vi "Load Sound Player.vi"(10 "Select sound player:":T1=1 items=["Sound Card", "Sound Visualizer"]) -> (0 "error out":errorcluster, 3 "Sound Player out":refnum<class "Sound Player.lvclass">)   [LabVIEW 2010, in "Sound Demo.lvclass"]
doc: "Dynamically load either Sound Visualizer or Sound Card.lvclass based on user input.\n\nBuild the path to the class using the string values of the Select sound player: ring control."
uses:
  Sound Demo.lvclass
  Select Sound Player.ctl
  Sound Player/Sound Player.lvclass
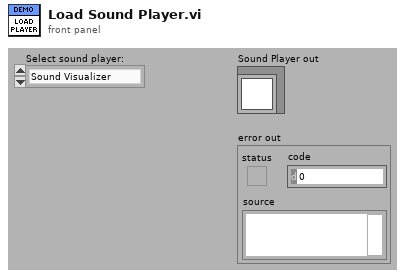
[diagram p1: front panel]
types:
  T1 = typedef "Sound Demo.lvclass/Select Sound Player.ctl" = u16
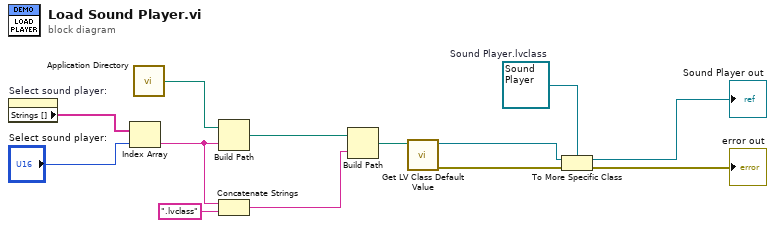
[diagram p0: block diagram]
diagram:
  w10 = refnum<class "Sound Player.lvclass"> refnum  # Sound Player.lvclass
  n1 = property on="Select sound player:" class="Ring (strict)"() -> ("Strings []"=w7:string[])  [unwired: 2 in, 2 out]
  n2 = Index Array "Index Array"(array=w7, index="Select sound player:") -> (element=w1:string)
  n3 = call <vilib>:"Application Directory.vi"() -> ("Application Directory"=w4:path)
  n4 = Build Path(base path=w4, name or relative path=w1) -> (appended path=w2:path)
  n5 = Concatenate Strings "Concatenate Strings"(w1, ".lvclass" ("string")) -> (w3:string)
  n6 = Build Path(base path=w2, name or relative path=w3) -> (appended path=w13:path)
  n7 = call <vilib>:"Get LV Class Default Value.vi"("class path"=w13) -> ("error out"=w11:errorcluster, "object"=w12:refnum<class>)  [unwired: 9 in]
  n8 = To More Specific Class(target class=w10, reference=w12, error in=w11) -> (specific class reference=→"Sound Player out":refnum<class "Sound Player.lvclass">, error out=→"error out":errorcluster)
